vi "change_position.vi"() -> ()   [LabVIEW 2021]
doc: "本VI是为《我和LabVIEW》一书编写的示例。\n关于本书的介绍请参考网页：\nhttp://ruanqizhen.spaces.live.com/blog/cns!5852D4F797C53FB6!4310.entry"
panel:
  in  "change my posistion":string
  in  "source右侧的控件":i32(slide) scale=0.0..100.0
  in  "exit":bool
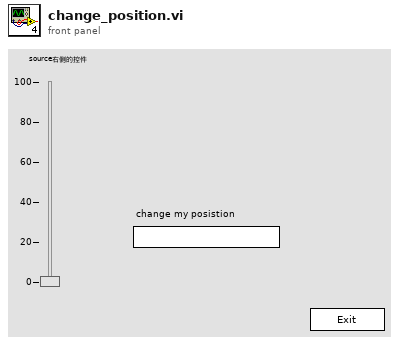
[diagram p1: front panel]
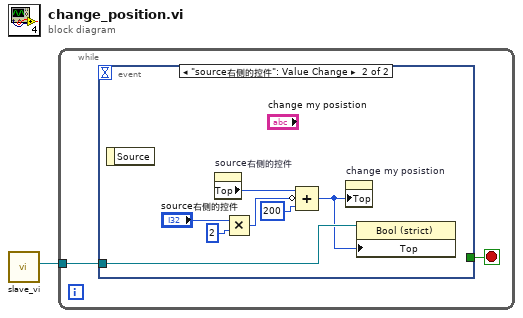
[diagram p0: block diagram]
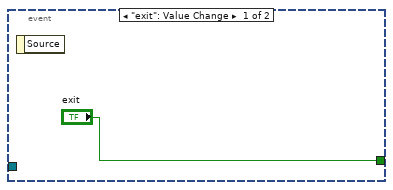
[diagram p2: hidden frame]
diagram:
  n1 = call "slave_vi.vi"() -> ("ref to control on another VI"=w1:refnum<vi>)  [unwired: 11 in]
  n2 = while {
    tunnel: w1 -> [w2]
    stop <- w3 stop-if-true
    n3 = event shown="[1] \"source右侧的控件\": Value Change" {
      selector: _ -> [_ _]
      dyn-events: _ -> [_ _]
      timeout: _ -> [_ _]
      tunnel: ["exit" _] -> w3
      tunnel: w2 -> [_ w6]
      event "exit": Value Change {
        n4 = event-data() -> ()  [unwired: 2 out]
      }
      event "source右侧的控件": Value Change {
        n5 = event-data() -> ()  [unwired: 2 out]
        n6 = property on="source右侧的控件" class="Slide (strict)"() -> ("Top"=w11:i32)  [unwired: 2 in, 2 out]
        n7 = Multiply(x="source右侧的控件", y=2) -> (x*y=w8:i32)
        n8 = Compound Arithmetic op=ADD(w11, invert w8, 200 ("值")) -> (w5:i32)
        n9 = property on="change my posistion" class="Str"("Top"=w5) -> ()  [unwired: 2 in, 2 out]
        n10 = property on="Property Node" class="Bool (strict)"(reference=w6, "Top"=w5) -> ()  [unwired: 1 in, 2 out]
      }
    }
  }
